vi "Cross Porticullis Drivetrain.vi"(11 "Local in":T1) -> (0 "Global Machine":T2, 3 "Local Machine":T1, 6 "Reset Enconder":bool)   [LabVIEW 2015]
uses:
  Type Defs/Porticullis State.ctl
  Type Defs/Intake State.ctl
  Robot Global Data.vi
panel:
  in  "Arm Height":dbl
  in  "Distancia da segunda reta":dbl=4.41 format="%#_13g"
  in  "Velocidade da segunda reta":dbl=0.7 format="%#_13g"
  in  "Velocidade da primeira re":dbl=-0.1 format="%#_13g"
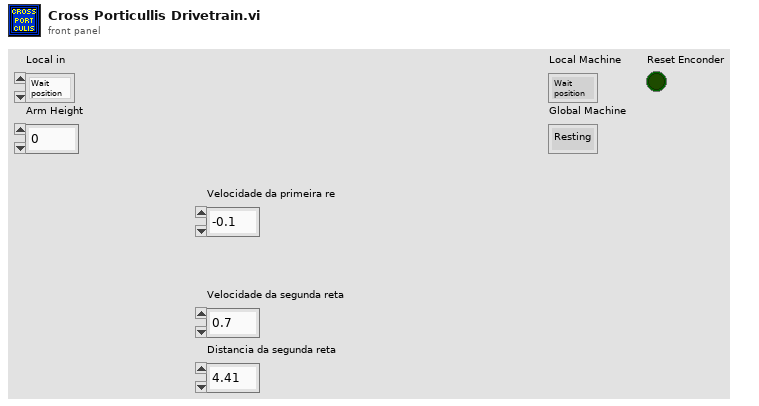
[diagram p1: front panel]
types:
  T1 = typedef "Porticullis State.ctl" = enum16{"Wait position", "Back up", "Reset Encoder", "Go Forward", "Finished"}
  T2 = typedef "Intake State.ctl" = enum16{"Resting", "Intake position", "Track Forward", "Raise Arm", "Track Reverse", "Defense position", "Armless Intake", "Cross Porticullis"}
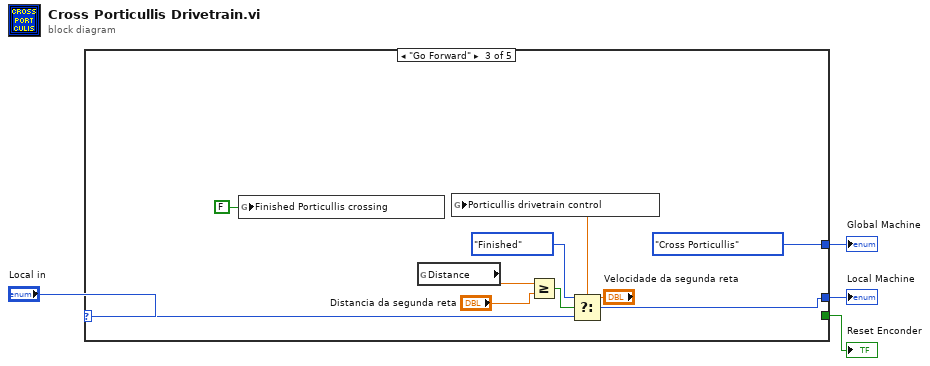
[diagram p0: block diagram]
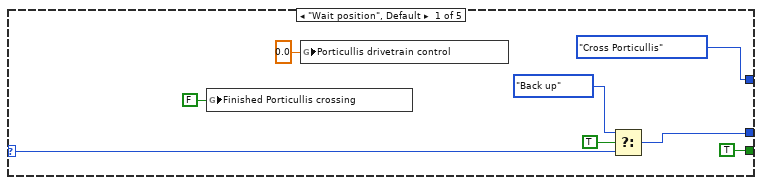
[diagram p2: hidden frame]
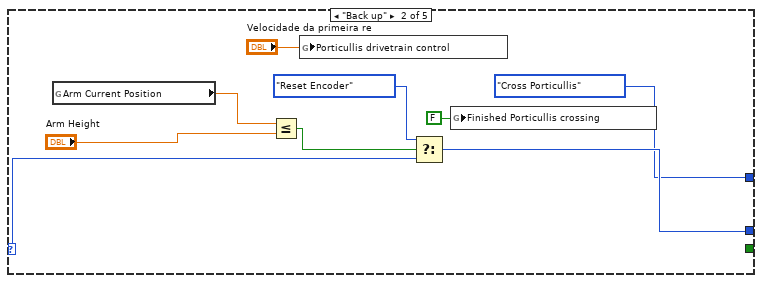
[diagram p3: hidden frame]
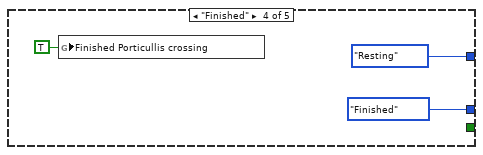
[diagram p4: hidden frame]
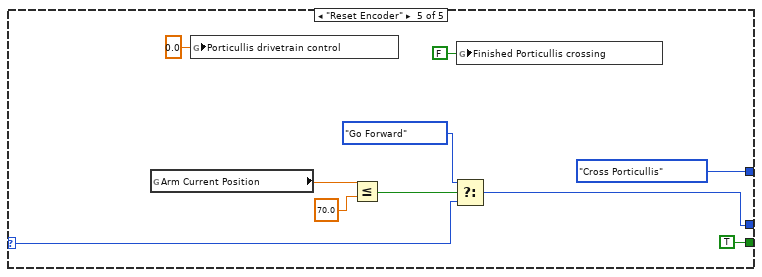
[diagram p5: hidden frame]
diagram:
  n1 = case shown="\"Go Forward\"" "Local in" {
    selector: "Local in" -> [w11 w18 w26 _ w35]
    tunnel: [w12 w19 w27 Porticullis_State."Finished" w37] -> w4
    tunnel: [Intake_State."Cross Porticullis" Intake_State."Cross Porticullis" Intake_State."Cross Porticullis" Intake_State."Resting" Intake_State."Cross Porticullis"] -> w3
    tunnel: [TRUE ("Crossing Porticullis?") _ _ _ TRUE ("Crossing Porticullis?")] -> w1
    frame "Wait position", Default {
      n2 = global write "Robot Global Data.vi" "Finished Porticullis crossing"(FALSE ("Finished Porticullis crossing")) -> ()
      n3 = global write "Robot Global Data.vi" "Porticullis drivetrain control"(0.0 ("Porticullis drivetrain control")) -> ()
      n4 = Select(t=Porticullis_State."Back up", s=TRUE, f=w11) -> (s? t:f=w12:T1)
    }
    frame "Back up" {
      n5 = global read "Robot Global Data.vi" "Arm Current Position"() -> (w21:dbl)
      n6 = Less Or Equal?(x=w21, y="Arm Height") -> (x <= y?=w20:bool)
      n7 = global write "Robot Global Data.vi" "Porticullis drivetrain control"("Velocidade da primeira re") -> ()
      n8 = Select(t=Porticullis_State."Reset Encoder", s=w20, f=w18) -> (s? t:f=w19:T1)
      n9 = global write "Robot Global Data.vi" "Finished Porticullis crossing"(FALSE ("Finished Porticullis crossing")) -> ()
    }
    frame "Go Forward" {
      n10 = global write "Robot Global Data.vi" "Finished Porticullis crossing"(FALSE ("Finished Porticullis crossing")) -> ()
      n11 = global read "Robot Global Data.vi" "Distance"() -> (w29:dbl)
      n12 = global write "Robot Global Data.vi" "Porticullis drivetrain control"("Velocidade da segunda reta") -> ()
      n13 = Greater Or Equal?(x=w29, y="Distancia da segunda reta") -> (x >= y?=w24:bool)
      n14 = Select(t=Porticullis_State."Finished", s=w24, f=w26) -> (s? t:f=w27:T1)
    }
    frame "Finished" {
      n15 = global write "Robot Global Data.vi" "Finished Porticullis crossing"(TRUE ("Finished Porticullis crossing")) -> ()
    }
    frame "Reset Encoder" {
      n16 = global read "Robot Global Data.vi" "Arm Current Position"() -> (w40:dbl)
      n17 = global write "Robot Global Data.vi" "Porticullis drivetrain control"(0.0 ("Porticullis drivetrain control")) -> ()
      n18 = Less Or Equal?(x=w40, y=70.0) -> (x <= y?=w38:bool)
      n19 = Select(t=Porticullis_State."Go Forward", s=w38, f=w35) -> (s? t:f=w37:T1)
      n20 = global write "Robot Global Data.vi" "Finished Porticullis crossing"(FALSE ("Finished Porticullis crossing")) -> ()
    }
  }
  "Local Machine" <- w4
  "Global Machine" <- w3
  "Reset Enconder" <- w1
